vi "Connect to Laser_Dx_client.vi"(0 "Laser IP Number":string="10.10.100.130", 1 "error in (no error)":errorcluster) -> (2 "Laser_Dx":refnum<k7>, 3 "error out":errorcluster, 4 "Channel":i64)   [LabVIEW 2020]
uses:
  Anemometry/Anemometry Sub Vis/Globals/LDA_global.vi
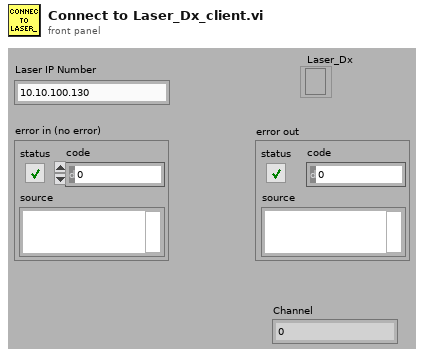
[diagram p1: front panel]
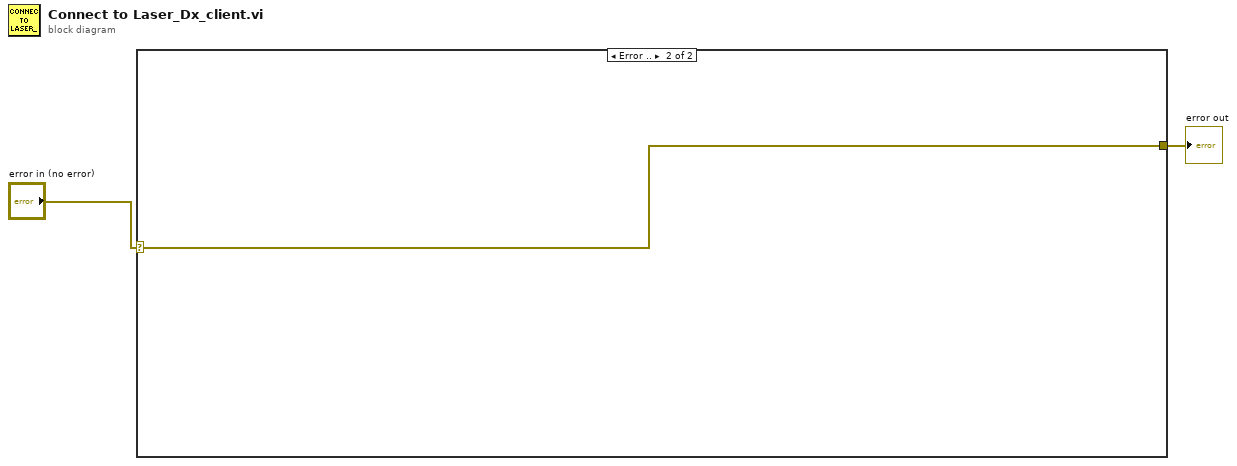
[diagram p0: block diagram]
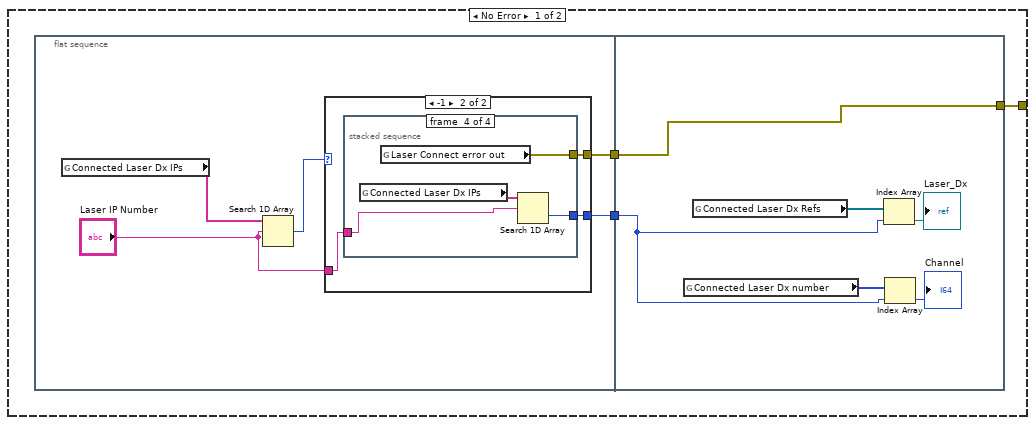
[diagram p2: hidden frame]
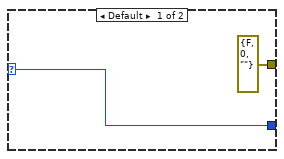
[diagram p3: hidden frame]
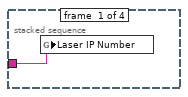
[diagram p4: hidden frame]
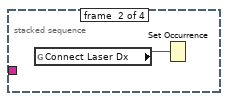
[diagram p5: hidden frame]
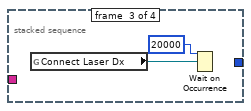
[diagram p6: hidden frame]
diagram:
  n1 = case shown="Error .." "error in (no error)" {
    selector: "error in (no error)" -> [_ w30]
    tunnel: [w3 w30] -> w2
    frame No Error {
      n2 = flat-sequence {
        tunnel: [w7] -> w5
        tunnel: [w6] -> w4
        tunnel: w5 -> [w27]
        tunnel: w4 -> [w24]
        tunnel: [w24] -> w3
        frame #0 {
          n3 = global read "LDA_global.vi" "Connected Laser Dx IPs"() -> (w8:string[])
          n4 = Search 1D Array(1D array=w8, element="Laser IP Number") -> (index of element=w9:i32)  [unwired: 1 in]
          n5 = case shown="-1" w9 {
            selector: w9 -> [w12 _]
            tunnel: "Laser IP Number" -> [_ w15]
            tunnel: [w12 w14] -> w7
            tunnel: [errorcluster {"status"=FALSE, "code"=0, "source"=""} ("Laser Connect error out") w13] -> w6
            frame Default {
            }
            frame -1 {
              n6 = stacked-sequence {
                tunnel: w15 -> [w16 _ _ w21]
                tunnel: [_ _ _ w22] -> w14
                tunnel: [_ _ _ w20] -> w13
                frame #0 {
                  n7 = global write "LDA_global.vi" "Laser IP Number"(w16) -> ()
                }
                frame #1 {
                  n8 = global read "LDA_global.vi" "Connect Laser Dx"() -> (w17:refnum<k4>)
                  n9 = Set Occurrence(w17) -> ()
                }
                frame #2 {
                  n10 = global read "LDA_global.vi" "Connect Laser Dx"() -> (w19:refnum<k4>)
                  n11 = Wait on Occurrence(2:w19, 3:20000 ("ms timeout (-1)")) -> ()  [unwired: 2 out]
                }
                frame #3 {
                  n12 = global read "LDA_global.vi" "Connected Laser Dx IPs"() -> (w23:string[])
                  n13 = global read "LDA_global.vi" "Laser Connect error out"() -> (w20:errorcluster)
                  n14 = Search 1D Array(1D array=w23, element=w21) -> (index of element=w22:i32)  [unwired: 1 in]
                }
              }
            }
          }
        }
        frame #1 {
          n15 = global read "LDA_global.vi" "Connected Laser Dx number"() -> (w28:i64[])
          n16 = global read "LDA_global.vi" "Connected Laser Dx Refs"() -> (w29:refnum<k7>[])
          n17 = Index Array(array=w29, index=w27) -> (element=→"Laser_Dx":refnum<k7>)
          n18 = Index Array(array=w28, index=w27) -> (element=→"Channel":i64)
        }
      }
    }
    frame Error {
    }
  }
  "error out" <- w2
